vi "C8855-01_InitWrite.vi"(5 "TrgEdge":u8, 7 "ExtT":bool, 8 "Moni":bool, 9 "MP":u32, 10 "GT":i32) -> ()   [LabVIEW 2017]
panel:
  out "InitFN":string
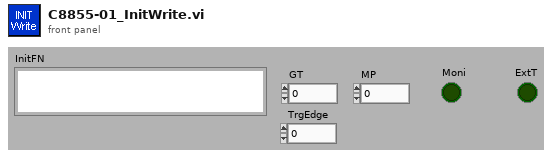
[diagram p1: front panel]
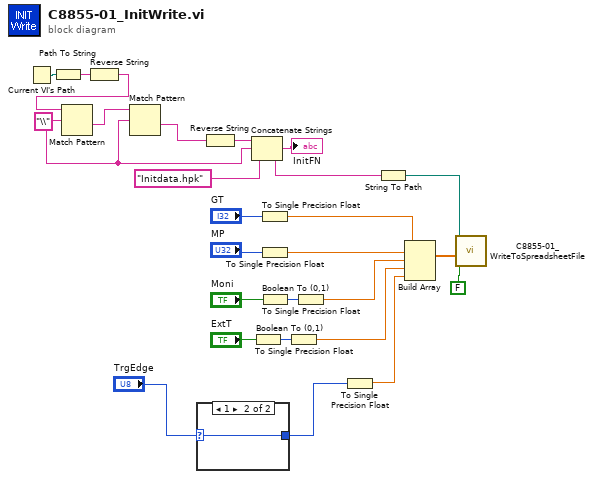
[diagram p0: block diagram]
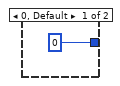
[diagram p2: hidden frame]
diagram:
  w17 = "\\" ("regular expression")
  n1 = Current VI's Path() -> (path=w25:path)
  n2 = Path To String(path=w25) -> (string=w24:string)
  n3 = Reverse String(1:w24) -> (0:w21:string)
  n4 = Match Pattern(string=w21, regular expression=w17) -> (after substring=w18:string)  [unwired: 4 out]
  n5 = Match Pattern(string=w18, regular expression=w17) -> (after substring=w23:string)  [unwired: 4 out]
  n6 = case shown="1" "TrgEdge" {
    selector: "TrgEdge" -> [_ w27]
    tunnel: [u8 0 w27] -> w1
    frame 0, Default {
    }
    frame 1 {
    }
  }
  n7 = Reverse String(1:w23) -> (0:w22:string)
  n8 = Concatenate Strings(w22, w17, "Initdata.hpk") -> (w19:string)
  "InitFN" <- w19
  n9 = Boolean To (0,1)(Boolean="ExtT") -> (0, 1=w5:i16)
  n10 = To Single Precision Float(number="GT") -> (single precision float=w13:sgl)
  n11 = To Single Precision Float(number="MP") -> (single precision float=w14:sgl)
  n12 = Boolean To (0,1)(Boolean="Moni") -> (0, 1=w11:i16)
  n13 = To Single Precision Float(number=w5) -> (single precision float=w4:sgl)
  n14 = To Single Precision Float(number=w11) -> (single precision float=w10:sgl)
  n15 = To Single Precision Float(number=w1) -> (single precision float=w3:sgl)
  n16 = String To Path(string=w19) -> (path=w7:path)
  n17 = Build Array(w13, w14, w10, w4, w3) -> (w8:sgl[])
  n18 = call "C8855-01_WriteToSpreadsheetFile.vi"("append to file? (new file:F)"=FALSE, "1D data"=w8, "file path (dialog if empty)"=w7) -> ()  [unwired: 4 in, 5 out]
